vi "ModifyGraph height.vi"(8 "error in (no error)":errorcluster, 10 "height (points) [256]":dbl=256.0, 11 "ITX Commands in":refnum<class "ITX Commands.lvclass">) -> (0 "error out":errorcluster, 3 "ITX Commands out":refnum<class "ITX Commands.lvclass">)   [LabVIEW 2016, in "ITX Commands.lvclass"]
uses:
  ITX Commands.lvclass
  ITX Commands.lvclass/ITX Commands.ctl
panel:
  out "resulting string":string
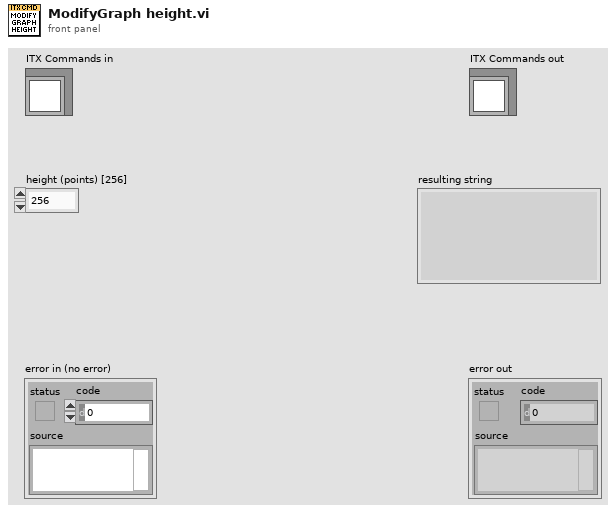
[diagram p1: front panel]
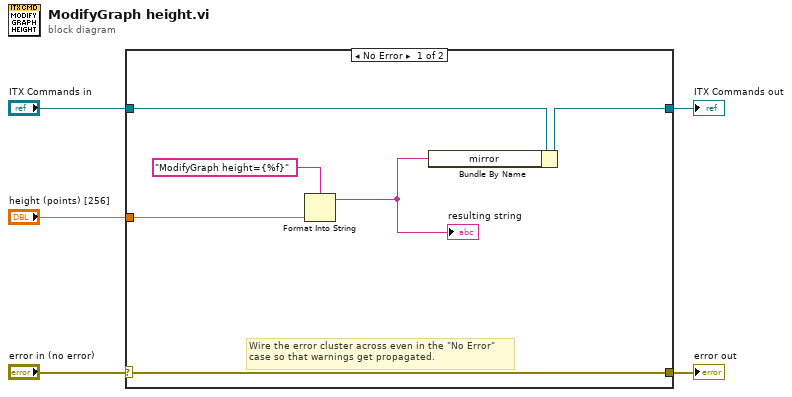
[diagram p0: block diagram]
diagram:
  n1 = case shown="No Error" "error in (no error)" {
    selector: "error in (no error)" -> [w11 w13]
    tunnel: [w11 w13] -> w4
    tunnel: [w7 w12] -> w2
    tunnel: "ITX Commands in" -> [w8 w12]
    tunnel: "height (points) [256]" -> [w6 _]
    frame No Error {
      # "Wire the error cluster across even in the \"No Error\"\ncase so that warnings get propagated."
      n2 = Format Into String(format string="ModifyGraph height={%f}", w6) -> (resulting string=w9:string)  [unwired: 2 in, 1 out]
      "resulting string" <- w9
      n3 = Bundle By Name(cluster=w8, "mirror"=w9) -> (w7:refnum<class "ITX Commands.lvclass">)
    }
    frame Error {
    }
  }
  "error out" <- w4
  "ITX Commands out" <- w2
